vi "Clear-object.vi"(8 "error in (no error)":errorcluster, 11 "Panes in":T1) -> (0 "error out":errorcluster, 3 "Panes out":T1)   [LabVIEW 2013, in "CameraVision.lvlib" / "CV-Panes.lvclass"]
uses:
  CV-Panes.lvclass
  Object-reference.ctl
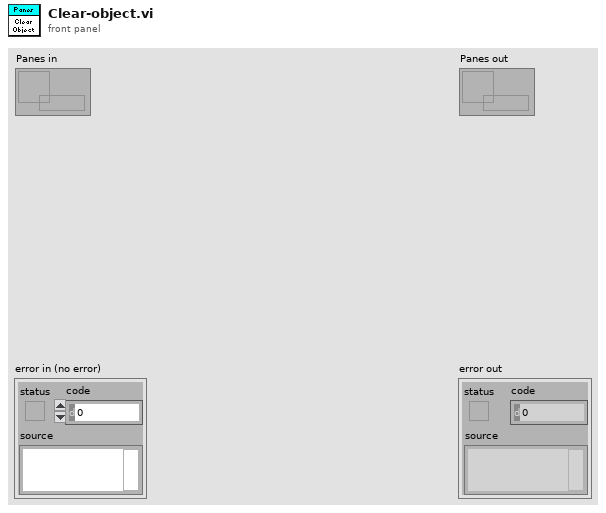
[diagram p1: front panel]
types:
  T1 = typedef "CameraVision.lvlib/CV-Panes.lvclass/Object-reference.ctl" = refnum<data-value>
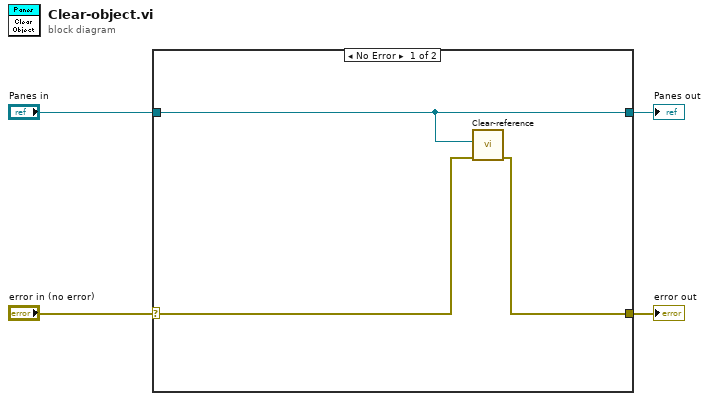
[diagram p0: block diagram]
diagram:
  n1 = case shown="No Error" "error in (no error)" {
    selector: "error in (no error)" -> [w5 w8]
    tunnel: [w7 w8] -> w3
    tunnel: [w6 w9] -> w1
    tunnel: "Panes in" -> [w6 w9]
    frame No Error {
      n2 = call "Clear-reference.vi"("error in (no error)"=w5, "Panes reference"=w6) -> ("error out"=w7:errorcluster)  [unwired: 8 in, 1 out]
    }
    frame Error {
    }
  }
  "error out" <- w3
  "Panes out" <- w1
